vi "WriteAimingBeamSetting.vi"(8 "error in":errorcluster, 11 "Aiming Beam Cluster":T1={"Aiming Beam COM Port"="COM3", "Min Current"=0.0, "Max Current"=63.0, "Default Current"=20.0, "Frequency(Hz)"=0}) -> (0 "error out":errorcluster)   [LabVIEW 2019]
uses:
  AimingBeam.ctl
  <vilib>/addons/_JKI.lib/Serialization/JSON/JKI JSON Serialization.lvlib
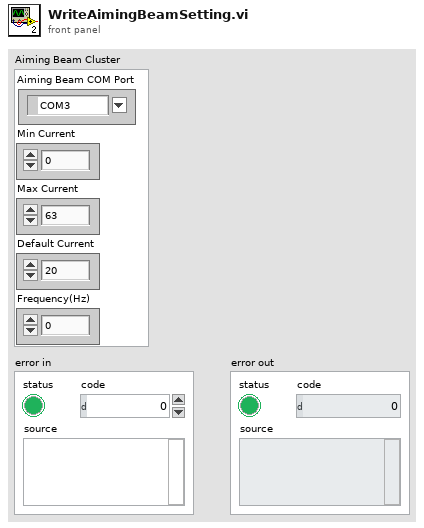
[diagram p1: front panel]
types:
  T1 = typedef "AimingBeam.ctl" = cluster{"Aiming Beam COM Port":refnum<visa-resource-name>, "Min Current":dbl, "Max Current":dbl, "Default Current":dbl, "Frequency(Hz)":u32}
  T2 = cluster{"Aiming Beam COM Port":string, "Min Current":dbl, "Max Current":dbl, "Default Current":dbl, "Frequency(Hz)":u32}
  T3 = enum16{"open", "replace", "create", "open or create", "replace or create", "replace or create with confirmation"}
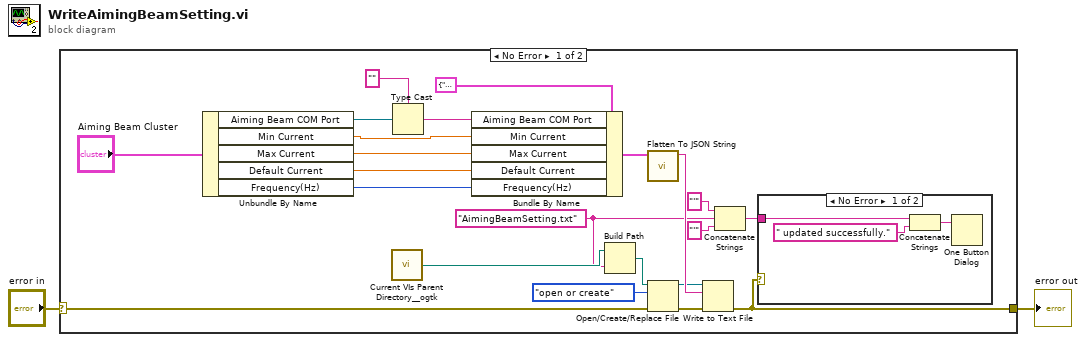
[diagram p0: block diagram]
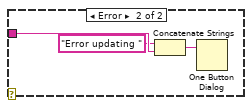
[diagram p2: hidden frame]
diagram:
  n1 = case shown="No Error" "error in" {
    selector: "error in" -> [w18 w31]
    tunnel: [w7 w31] -> w2
    frame No Error {
      w6 = "AimingBeamSetting.txt"
      n2 = Unbundle By Name("Aiming Beam Cluster") -> ("Aiming Beam COM Port"=w16:refnum<visa-resource-name>, "Min Current"=w14:dbl, "Max Current"=w13:dbl, "Default Current"=w12:dbl, "Frequency(Hz)"=w11:u32)
      n3 = call <userlib>:"Current VIs Parent Directory__ogtk.vi"() -> ("Parent Directory (+ Relative)"=w24:path)  [unwired: 5 in]
      n4 = Type Cast(type="", x=w16) -> (*(type *) &x=w9:string)
      n5 = Bundle By Name(cluster=T2 {"Aiming Beam COM Port"="", "Min Current"=0.0, "Max Current"=63.0, "Default Current"=20.0, "Frequency(Hz)"=0}, "Aiming Beam COM Port"=w9, "Min Current"=w14, "Max Current"=w13, "Default Current"=w12, "Frequency(Hz)"=w11) -> (w10:T2)
      n6 = Build Path(base path=w24, name or relative path=w6) -> (appended path=w23:path)
      n7 = call <vilib>:"Flatten To JSON String.vi"("Variant"=w10) -> ("JSON String"=w21:string)  [unwired: 9 in, 1 out]
      n8 = Open/Create/Replace File(file path (use dialog)=w23, error in=w18, operation (0:open)=T3."open or create") -> (refnum out=w20:refnum<file>, error out=w19:errorcluster)  [unwired: 3 in, 1 out]
      n9 = Write to Text File(file (use dialog)=w20, text=w21, error in=w19) -> (error out=w7:errorcluster)  [unwired: 1 in, 2 out]
      n10 = Concatenate Strings("'" ("string"), w6, "'" ("string")) -> (w3:string)
      n11 = case shown="No Error" w7 {
        tunnel: w3 -> [w27 w29]
        frame No Error {
          n12 = Concatenate Strings(w27, " updated successfully." ("string")) -> (w25:string)
          n13 = One Button Dialog(message=w25) -> ()  [unwired: 1 in, 1 out]
        }
        frame Error {
          n14 = Concatenate Strings("Error updating " ("string"), w29) -> (w30:string)
          n15 = One Button Dialog(message=w30) -> ()  [unwired: 1 in, 1 out]
        }
      }
    }
    frame Error {
    }
  }
  "error out" <- w2
